vi "run.vi"(7 "abortEvent":refnum<user-event>, 8 "error in (no error)":errorcluster, 10 "TestResult in":refnum<class "TestResult.lvclass">, 11 "TestSuite in":refnum<class "TestSuite.lvclass">) -> (0 "error out":errorcluster, 2 "TestResult out":refnum<class "TestResult.lvclass">, 3 "TestSuite out":refnum<class "TestSuite.lvclass">)   [LabVIEW 2013, in "TestSuite.lvclass"]
uses:
  TestSuite.lvclass
  TestResult/TestResult.lvclass
  TestSuite.lvclass/TestSuite.ctl
  Method--enum.ctl
  suiteStatusChanged--Cluster.ctl
  suiteStatus--enum.ctl
  TestCase/TestCase.lvclass
  Libraries/VITesterUtilities.lvlib
panel:
  # "JKI VI Tester for LabVIEW\nhttp://jkisoft.com/vi-tester\nCopyright (C) 2007-2009, JKI <info@jkisoft.com>\nALL RIGHTS RESERVED"
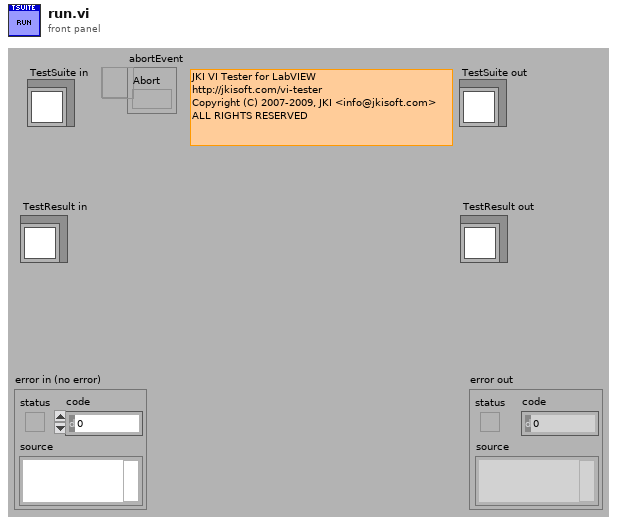
[diagram p1: front panel]
types:
  T1 = typedef "TestSuite.lvclass/suiteStatusChanged--Cluster.ctl" = cluster{"TestSuite":refnum<class>, "suiteStatus":T2}
  T2 = typedef "TestSuite.lvclass/suiteStatus--enum.ctl" = enum16{"suiteStart", "suiteStop", "suiteSkip"}
  T3 = typedef "TestSuite.lvclass/Method--enum.ctl" = enum16{"setUp", "tearDown"}
  T4 = typedef "TestResult.lvclass/shouldStop.ctl" = bool
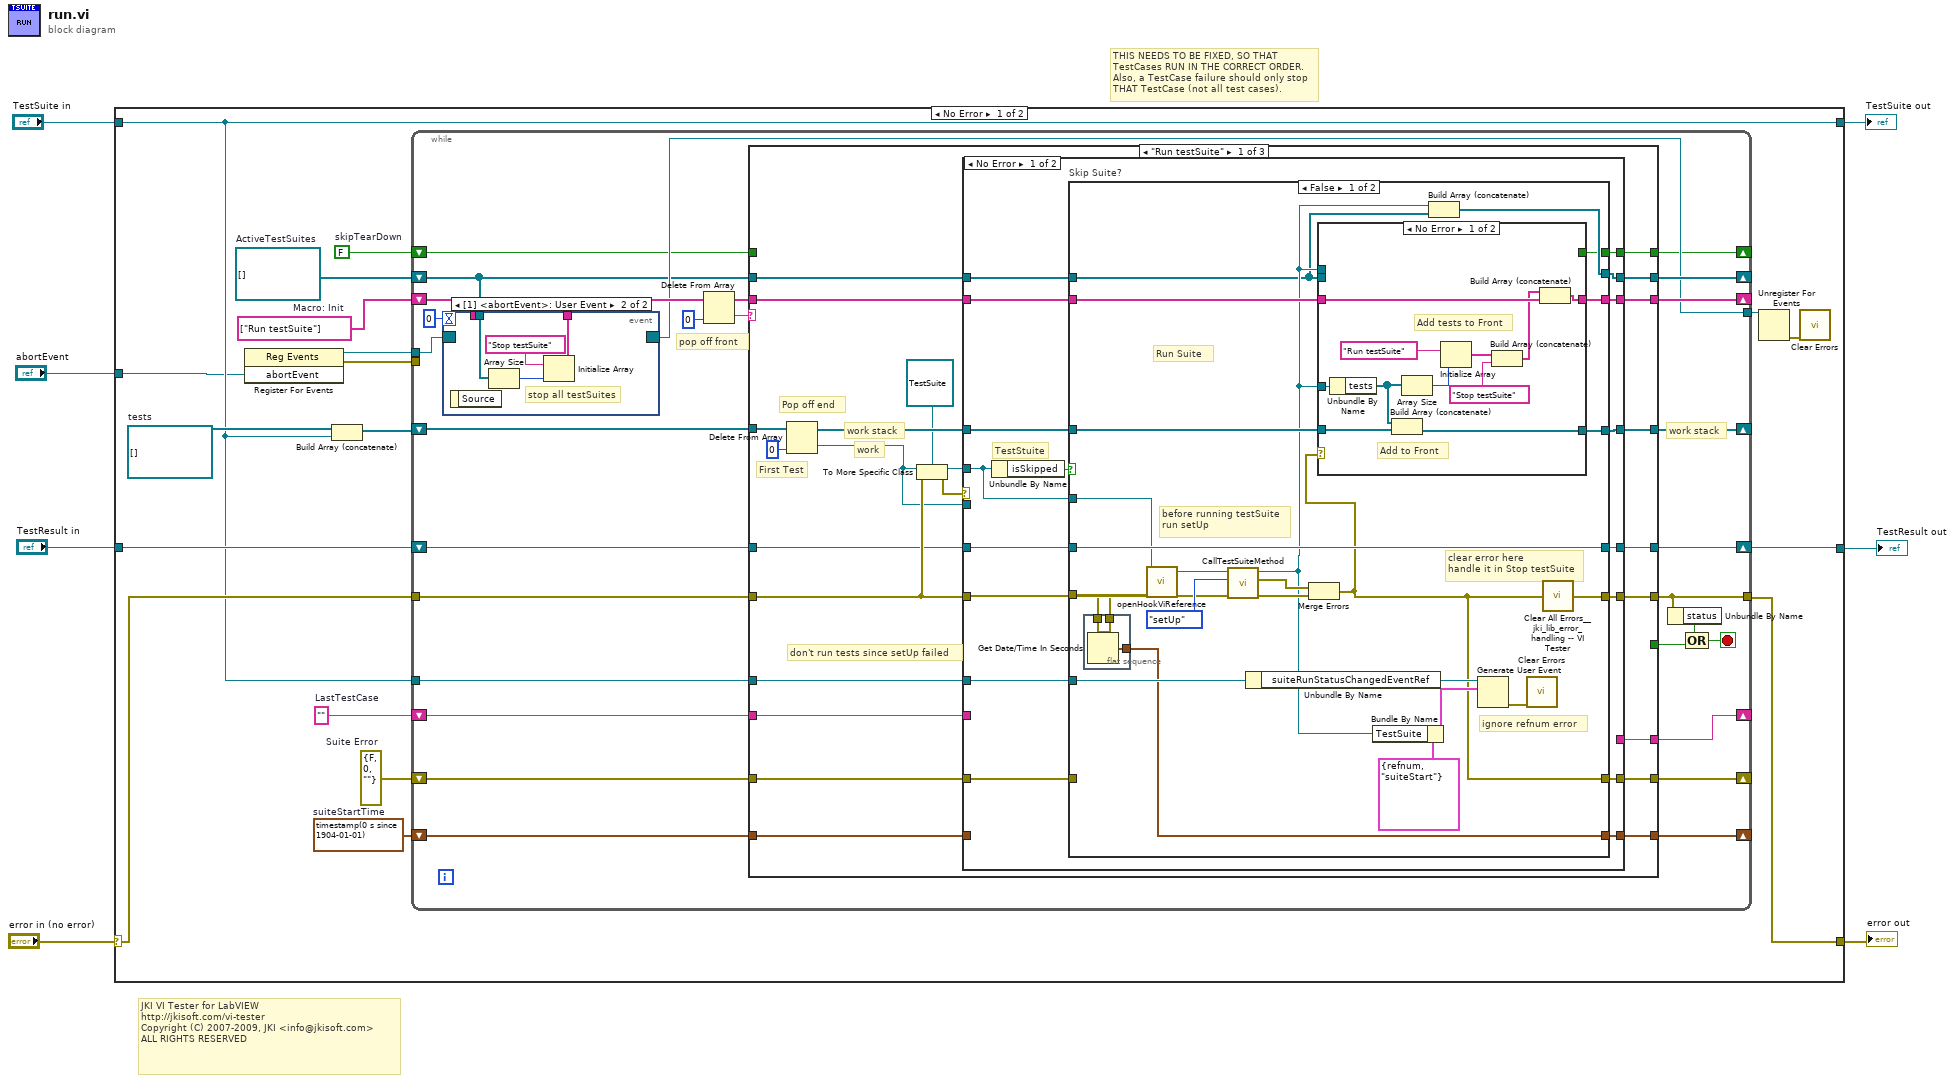
[diagram p0: block diagram]
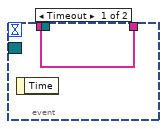
[diagram p2: hidden frame]
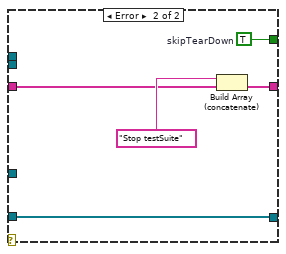
[diagram p3: hidden frame]
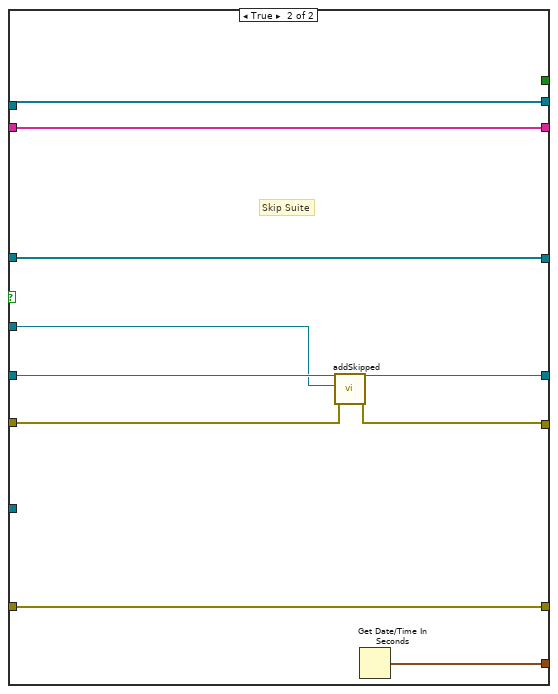
[diagram p4: hidden frame]
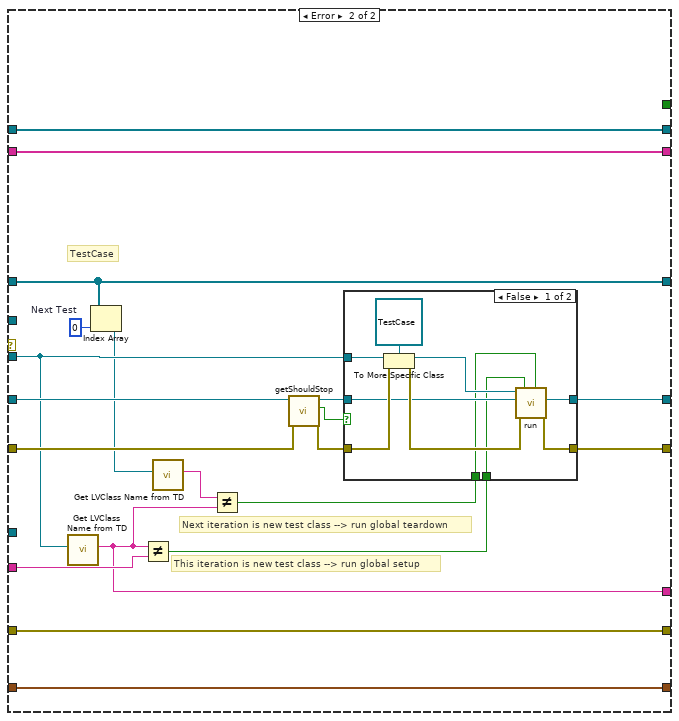
[diagram p5: hidden frame]
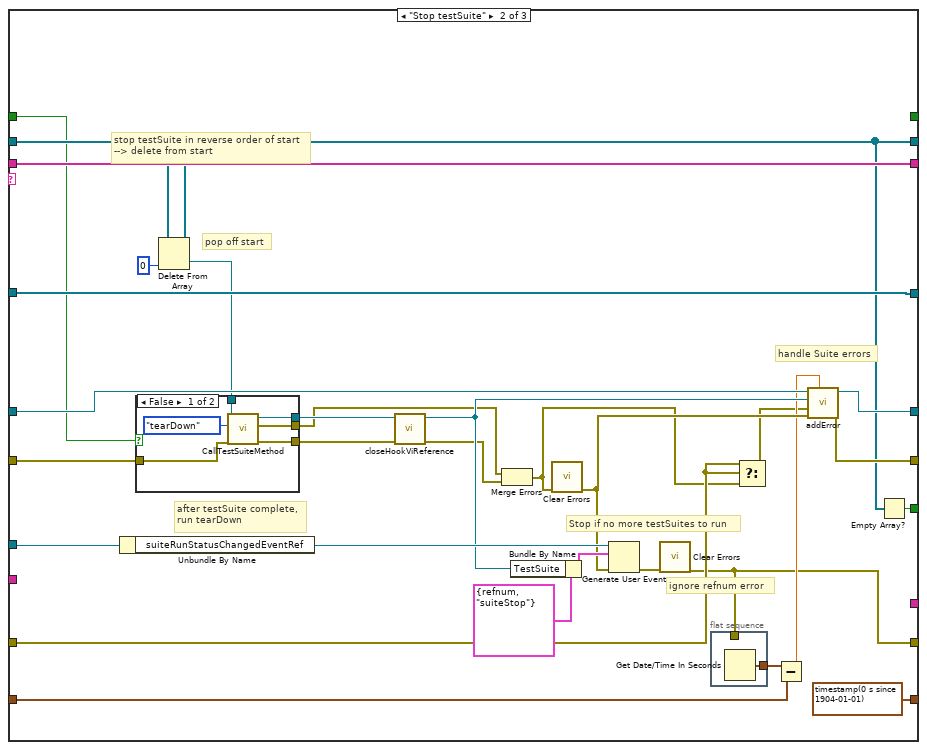
[diagram p7: hidden frame]
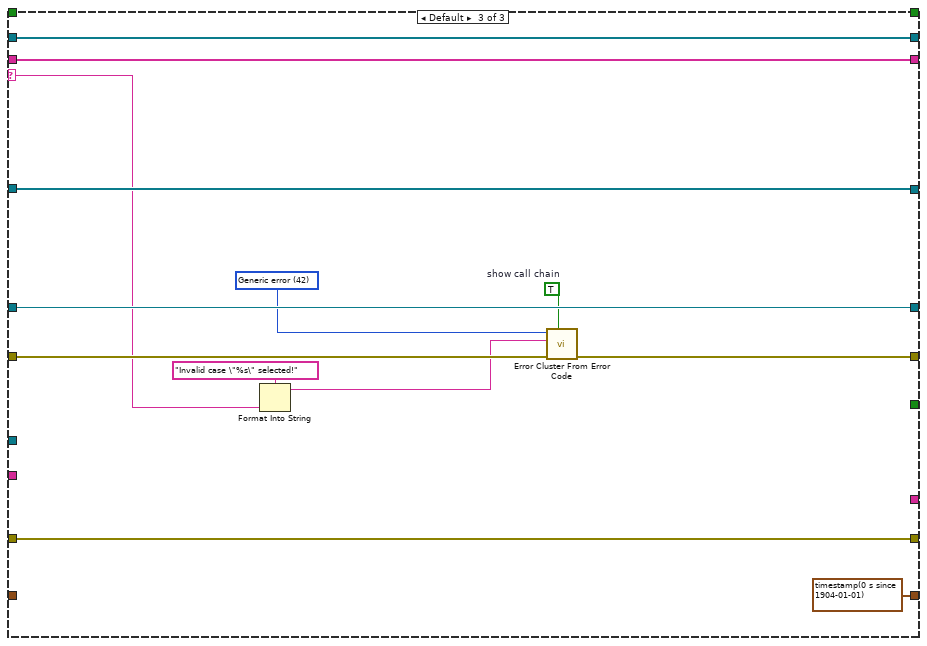
[diagram p9: hidden frame]
diagram:
  # "JKI VI Tester for LabVIEW\nhttp://jkisoft.com/vi-tester\nCopyright (C) 2007-2009, JKI <info@jkisoft.com>\nALL RIGHTS RESERVED"
  # "THIS NEEDS TO BE FIXED, SO THAT TestCases RUN IN THE CORRECT ORDER.  Also, a TestCase failure should only stop THAT TestCase (not all test cases)."
  n1 = case shown="No Error" "error in (no error)" {
    selector: "error in (no error)" -> [w21 w241]
    tunnel: [w20 w241] -> w6
    tunnel: [w17 w240] -> w4
    tunnel: "TestSuite in" -> [w17 w240]
    tunnel: "TestResult in" -> [w22 w239]
    tunnel: [w19 w239] -> w2
    tunnel: "abortEvent" -> [w16 _]
    frame No Error {
      w8 = ""  # LastTestCase
      w9 = errorcluster {"status"=FALSE, "code"=0, "source"=""}  # Suite Error
      w10 = timestamp(0 s since 1904-01-01)  # suiteStartTime
      w18 = string[] ["Run testSuite"]  # Macro: Init
      w24 = refnum<class>[] []  # tests
      w25 = refnum<class "TestSuite.lvclass">[] []  # ActiveTestSuites
      w11 = FALSE  # skipTearDown
      n2 = register-events(w16) -> (reference out=w14:refnum<event-registration>, error out=w15:errorcluster)  [unwired: 2 in]
      n3 = Build Array (concatenate)(w24, w17) -> (w23:refnum<class>[])
      n4 = while {
        tunnel: w21 -> [w54]
        tunnel: [w35] -> w20
        shift-right: [w52] -> _
        shift-left: w23 -> [w53]
        shift-right: [w51] -> w19
        shift-left: w22 -> [w50]
        shift-right: [w47] -> _
        shift-left: w18 -> [w41]
        shift-right: [w46] -> _
        shift-left: w25 -> [w38]
        tunnel: w17 -> [w44]
        tunnel: w15 -> [_]
        tunnel: w14 -> [w43]
        tunnel: [w39] -> w13
        shift-right: [w37] -> _
        shift-left: w11 -> [w36]
        shift-right: [w31] -> _
        shift-left: w10 -> [w30]
        shift-right: [w28] -> _
        shift-left: w9 -> [w29]
        shift-right: [w26] -> _
        shift-left: w8 -> [w27]
        stop <- w32 stop-if-true
        # "pop off front"
        # "work stack"
        n5 = event shown="[1] <abortEvent>: User Event" {
          selector: w43 -> [_ _]
          dyn-events: [_ _] -> w39
          timeout: 0 -> [_ _]
          tunnel: w41 -> [w55 _]
          tunnel: [w55 w56] -> w40
          tunnel: w38 -> [_ w57]
          event Timeout {
            n6 = event-data() -> ()  [unwired: 1 in, 1 out]
          }
          event User Event {
            # "stop all testSuites"
            n7 = event-data() -> ()  [unwired: 1 in, 1 out]
            n8 = Array Size(array=w57) -> (size(s)=w58:i32)
            n9 = Initialize Array("Stop testSuite", w58) -> (w56:string[])
          }
        }
        n10 = Delete From Array(array=w40, index=0) -> (deleted portion=w49:string, array with subset deleted=w48:string[])  [unwired: 1 in]
        n11 = case "TestSuite Action" shown="\"Run testSuite\"" w49 {
          selector: w49 -> [_ _ w231]
          tunnel: w54 -> [w83 w215 w233]
          tunnel: [w82 w214 w232] -> w35
          tunnel: w53 -> [w81 w212 w236]
          tunnel: [w78 w212 w236] -> w52
          tunnel: [w77 w213 w235] -> w51
          tunnel: w50 -> [w76 w216 w235]
          tunnel: w38 -> [w69 w210 w238]
          tunnel: w48 -> [w70 w211 w237]
          tunnel: [w71 w211 w237] -> w47
          tunnel: [w68 w207 w238] -> w46
          tunnel: [_ w208 _] -> w33
          tunnel: w44 -> [w67 w203 _]
          tunnel: w36 -> [_ w194 _]
          tunnel: [w66 _ _] -> w37
          tunnel: [w65 timestamp(0 s since 1904-01-01) ("suiteStartTime") timestamp(0 s since 1904-01-01) ("suiteStartTime")] -> w31
          tunnel: w30 -> [w64 w192 _]
          tunnel: w29 -> [w63 w189 w226]
          tunnel: [w62 w186 w226] -> w28
          tunnel: w27 -> [w61 _ _]
          tunnel: [w60 _ _] -> w26
          frame "Run testSuite" {
            # "don't run tests since setUp failed"
            # "First Test"
            # "Pop off end"
            # "work"
            # "work stack"
            n12 = Delete From Array(array=w81, index=0) -> (deleted portion=w80:refnum<class>, array with subset deleted=w79:refnum<class>[])  [unwired: 1 in]
            n13 = To More Specific Class(target class=refnum<class "TestSuite.lvclass"> refnum ("TestSuite out"), reference=w80, error in=w83) -> (specific class reference=w73:refnum<class "TestSuite.lvclass">, error out=w74:errorcluster)
            n14 = case shown="No Error" w74 {
              tunnel: [w96 w172] -> w77
              tunnel: [w97 w173] -> w82
              tunnel: w80 -> [_ w158]
              tunnel: w83 -> [w90 w169]
              tunnel: [w99 w160] -> w78
              tunnel: w79 -> [w100 w160]
              tunnel: w73 -> [w89 _]
              tunnel: w76 -> [w98 w171]
              tunnel: [w94 w166] -> w71
              tunnel: w70 -> [w95 w166]
              tunnel: w69 -> [w93 w165]
              tunnel: [w92 w165] -> w68
              tunnel: w67 -> [w91 _]
              tunnel: [w87 _] -> w66
              tunnel: [w86 w164] -> w65
              tunnel: w64 -> [_ w164]
              tunnel: w63 -> [w85 w163]
              tunnel: [w84 w163] -> w62
              tunnel: w61 -> [_ w162]
              tunnel: [_ w154] -> w60
              frame No Error {
                # "TestStuite"
                n15 = Unbundle By Name(w89) -> ("isSkipped"=w88:bool)
                n16 = case "Skip Suite?" shown="False" w88 {
                  tunnel: w100 -> [w125 w151]
                  tunnel: [w124 w151] -> w99
                  tunnel: w98 -> [w122 w150]
                  tunnel: [w101 w147] -> w97
                  tunnel: [w122 w149] -> w96
                  tunnel: w95 -> [w111 w153]
                  tunnel: [w110 w153] -> w94
                  tunnel: w93 -> [w108 w152]
                  tunnel: [w107 w152] -> w92
                  tunnel: w91 -> [w121 _]
                  tunnel: w90 -> [w105 w146]
                  tunnel: w89 -> [w112 w148]
                  tunnel: [w106 _] -> w87
                  tunnel: [w103 w145] -> w86
                  tunnel: w85 -> [_ w144]
                  tunnel: [w102 w144] -> w84
                  frame False {
                    # "clear error here\nhandle it in Stop testSuite"
                    # "Run Suite"
                    # "ignore refnum error"
                    # "before running testSuite\nrun setUp"
                    n17 = flat-sequence {
                      tunnel: [w127] -> w104
                      tunnel: w105 -> [w127]
                      tunnel: [w126] -> w103
                      frame #0 {
                        n18 = Get Date/Time In Seconds() -> (seconds since 1Jan1904=w126:timestamp)
                      }
                    }
                    n19 = call "openHookViReference.vi"("error in (no error)"=w104, "TestSuite in"=w112) -> ("error out"=w117:errorcluster, "TestSuite out"=w116:refnum<class "TestSuite.lvclass">)  [unwired: 8 in]
                    n20 = call "CallTestSuiteMethod.vi"("error in"=w117, "method"=Method--enum."setUp", "TestSuite in"=w116) -> ("error out"=w114:errorcluster, "Test Method Error"=w115:errorcluster, "TestSuite out"=w109:refnum<class "TestSuite.lvclass">)  [unwired: 6 in]
                    n21 = Unbundle By Name(w121) -> ("suiteRunStatusChangedEventRef"=w120:refnum<user-event>)
                    n22 = Merge Errors(w115, w114) -> (w102:errorcluster)
                    n23 = case shown="No Error" w102 {
                      tunnel: w125 -> [w138 w143]
                      tunnel: [w137 w143] -> w124
                      tunnel: w109 -> [w131 _]
                      tunnel: w111 -> [w130 w141]
                      tunnel: [w128 w140] -> w110
                      tunnel: w109 -> [_ _]
                      tunnel: w108 -> [_ _]
                      tunnel: [_ w139] -> w106
                      frame No Error {
                        # "Add tests to Front"
                        # "Add to Front"
                        n24 = Unbundle By Name(w131) -> ("tests"=w135:refnum<class>[])
                        n25 = Build Array (concatenate)(w135, w138) -> (w137:refnum<class>[])
                        n26 = Array Size(array=w135) -> (size(s)=w134:i32)
                        n27 = Initialize Array("Run testSuite", w134) -> (w132:string[])
                        n28 = Build Array (concatenate)(w132, "Stop testSuite") -> (w129:string[])
                        n29 = Build Array (concatenate)(w129, w130) -> (w128:string[])
                      }
                      frame Error {
                        w139 = TRUE  # skipTearDown
                        n30 = Build Array (concatenate)("Stop testSuite", w141) -> (w140:string[])
                      }
                    }
                    n31 = Bundle By Name(cluster=T1 {"TestSuite"=refnum, "suiteStatus"=enum."suiteStart"} ("suiteStatusChanged"), "TestSuite"=w109) -> (w119:T1)
                    n32 = Build Array (concatenate)(w109, w108) -> (w107:refnum<class "TestSuite.lvclass">[])
                    n33 = Generate User Event(user event=w120, event data cluster=w119) -> (error out=w118:errorcluster)  [unwired: 2 in, 1 out]
                    n34 = call <vilib>:"Clear Errors.vi"("error in (no error)"=w118) -> ()  [unwired: 6 in, 1 out]
                    n35 = call "Clear All Errors__jki_lib_error_handling -- VI Tester.vi"("error in"=w102) -> ("no error out"=w101:errorcluster)  [unwired: 4 in]
                  }
                  frame True {
                    # "Skip Suite"
                    n36 = call-dynamic "addSkipped.vi"("error in (no error)"=w146, "test"=w148, "TestResult in"=w150) -> ("error out"=w147:errorcluster, "TestResult out"=w149:refnum<class "TestResult.lvclass">)  [unwired: 7 in]
                    n37 = Get Date/Time In Seconds() -> (seconds since 1Jan1904=w145:timestamp)
                  }
                }
              }
              frame Error {
                w159 = 0  # Next Test
                # "This iteration is new test class --> run global setup"
                # "Next iteration is new test class --> run global teardown"
                # "TestCase"
                n38 = call "Get LVClass Name from TD.vi"("Variant"=w158) -> ("LVClass Name"=w154:string)  [unwired: 9 in, 1 out]
                n39 = Index Array(array=w160, index=w159) -> (element=w157:refnum<class>)
                n40 = Not Equal?(x=w154, y=w162) -> (x != y?=w161:bool)
                n41 = call "Get LVClass Name from TD.vi"("Variant"=w157) -> ("LVClass Name"=w156:string)  [unwired: 9 in, 1 out]
                n42 = Not Equal?(x=w156, y=w154) -> (x != y?=w155:bool)
                n43 = call-dynamic "getShouldStop.vi"("error in (no error)"=w169, "TestResult in"=w171) -> ("error out"=w168:errorcluster, "shouldStop"=w167:T4, "TestResult out"=w170:refnum<class "TestResult.lvclass">)  [unwired: 7 in]
                n44 = case shown="False" w167 {
                  tunnel: w158 -> [w182 _]
                  tunnel: [w181 w184] -> w173
                  tunnel: [w180 w185] -> w172
                  tunnel: w170 -> [w176 w185]
                  tunnel: w168 -> [w179 w184]
                  tunnel: w161 -> [w175 _]
                  tunnel: w155 -> [w174 _]
                  frame False {
                    n45 = To More Specific Class(target class=refnum<class "TestCase.lvclass"> refnum ("reference in"), reference=w182, error in=w179) -> (specific class reference=w178:refnum<class "TestCase.lvclass">, error out=w177:errorcluster)
                    n46 = call "run.vi"("RunGlobalTearDown"=w174, "RunGlobalSetup"=w175, "error in (no error)"=w177, "TestResult in (None: Create New)"=w176, "TestCase in"=w178) -> ("error out"=w181:errorcluster, "TestResult out"=w180:refnum<class "TestResult.lvclass">)  [unwired: 4 in, 1 out]
                  }
                  frame True {
                  }
                }
              }
            }
          }
          frame "Stop testSuite" {
            # "handle Suite errors"
            # "ignore refnum error"
            # "pop off start"
            # "Stop if no more testSuites to run"
            # "stop testSuite in reverse order of start\n--> delete from start"
            # "after testSuite complete,\nrun tearDown"
            n47 = Unbundle By Name(w203) -> ("suiteRunStatusChangedEventRef"=w206:refnum<user-event>)
            n48 = Delete From Array(array=w210, index=0) -> (deleted portion=w209:refnum<class "TestSuite.lvclass">, array with subset deleted=w207:refnum<class "TestSuite.lvclass">[])  [unwired: 1 in]
            n49 = case shown="False" w194 {
              tunnel: w215 -> [w222 w225]
              tunnel: w209 -> [w221 w224]
              tunnel: [w220 w224] -> w201
              tunnel: [w219 w225] -> w199
              tunnel: [w218 w225] -> w198
              frame False {
                n50 = call "CallTestSuiteMethod.vi"("error in"=w222, "method"=Method--enum."tearDown", "TestSuite in"=w221) -> ("error out"=w219:errorcluster, "Test Method Error"=w218:errorcluster, "TestSuite out"=w220:refnum<class "TestSuite.lvclass">)  [unwired: 6 in]
              }
              frame True {
              }
            }
            n51 = call "closeHookViReference.vi"("error in (no error)"=w199, "TestSuite in"=w201) -> ("error out"=w197:errorcluster, "TestSuite out"=w200:refnum<class "TestSuite.lvclass">)  [unwired: 8 in]
            n52 = Merge Errors(w198, w197) -> (w188:errorcluster)
            n53 = Bundle By Name(cluster=T1 {"TestSuite"=refnum, "suiteStatus"=enum."suiteStop"} ("suiteStatusChanged"), "TestSuite"=w200) -> (w205:T1)
            n54 = call <vilib>:"Clear Errors.vi"("error in (no error)"=w188) -> ("error out"=w196:errorcluster)  [unwired: 6 in]
            n55 = Generate User Event(user event=w206, event data cluster=w205, error in=w196) -> (error out=w204:errorcluster)  [unwired: 1 in, 1 out]
            n56 = call <vilib>:"Clear Errors.vi"("error in (no error)"=w204) -> ("error out"=w186:errorcluster)  [unwired: 6 in]
            n57 = flat-sequence {
              tunnel: w186 -> [_]
              tunnel: [w217] -> w193
              frame #0 {
                n58 = Get Date/Time In Seconds() -> (seconds since 1Jan1904=w217:timestamp)
              }
            }
            n59 = Select(t=w189, s=w189, f=w188) -> (s? t:f=w187:errorcluster)
            n60 = Subtract(x=w193, y=w192) -> (x-y=w191:dbl)
            n61 = call-dynamic "addError.vi"("execution time (sec)"=w191, "error in (no error)"=w196, "test error"=w187, "test"=w200, "TestResult in"=w216) -> ("error out"=w214:errorcluster, "TestResult out"=w213:refnum<class "TestResult.lvclass">)  [unwired: 5 in]
            n62 = Empty Array?(array=w207) -> (empty?=w208:bool)
          }
          frame Default {
            w228 = TRUE  # show call chain
            w234 = 42 items=["No error", "Argument error", "Memory is full", "Out of zone", "End of file", "File already open", "Generic file I/O error", "File not found", "File permission error", "Disk is full", "Duplicate path", "Too many files open", "System feature not enabled", "Resource file not found", "Cannot add resource", "Resource not found", "Image not found", "Image memory error", "Pen does not exist", "Config type invalid", "Config token not found", "Config parse error", "Config memory error", "Bad external code format", "Bad external code offset", "External code not present", "Null window", "Destroy window error", "Null menu", "Print aborted", "Bad print record", "Print driver error", "Windows error during printing", "Memory error during printing", "Print dialog error", "Generic print error", "Invalid device refnum", "Device not found", "Device parameter error", "Device unit error", "Cannot open device", "Device call aborted", "Generic error", "Cancelled by user", "Object ID too low", "Object ID too high", "Object not in heap", "Unknown heap", "Unknown object (invalid DefProc)", "Unknown object (DefProc not in table)", "Message out of range", "Invalid (null) method", "Unknown message", "Manager call not supported", "Bad address", "Network operation in progress", "Network operation timed out", "Connection is busy", "Network attribute not supported", "Network error", "Address in use", "System out of memory", "Connection aborted", "Connection refused", "Not connected", "Already connected", "Connection closed", "Initialization error (interapplication manager)", "Bad occurrence", "Wait on unbound occurrence handler", "Occurrence queue overflow", "Datalog type conflict", "Unused", "Unrecognized type (interapplication manager)", "Memory corrupt", "Failed to make temporary DLL", "Old CIN version", "Drag socket not found", "Failed to load drop-object", "Failed to register OLE object", "Failed to release OLE object", "Format specifier type mismatch", "Unknown format specifier", "Too few format specifiers", "Too many format specifiers", "Scan failed", "Newer CIN version", "Error converting to variant", "Runtime menu error", "Password tampered", "Variant attribute not found", "Incompatible variant data type", "Event data is not available", "Event Store is not present", "Occurrence is not found", "Event Queue is not created", "Event info is not available", "Refnum passed is NULL", "Error retrieving Class GUID", "Error retrieving CoClass GUID", "Error retrieving TypeLib GUID.", "Bad built application magic bytes.", "Specific driver is different from the specific driver associated with the Logical Name.", "There is no session opened to the class driver.", "Max Error", "MAX - Error with config objects", "MAX - Error loading configuration", "MAX - Group not supported"]
            n63 = Format Into String(format string="Invalid case \"%s\" selected!", w231) -> (resulting string=w229:string)  [unwired: 2 in, 1 out]
            n64 = call <vilib>:"Error Cluster From Error Code.vi"("show call chain? (False)"=w228, "error in (no error)"=w233, "error message (\"\")"=w229, "error code (0)"=w234) -> ("error out"=w232:errorcluster)  [unwired: 5 in]
          }
        }
        n65 = Unbundle By Name(w35) -> ("status"=w34:bool)
        n66 = Compound Arithmetic op=OR(w34, w33) -> (w32:bool)
      }
      n67 = Unregister For Events(event registration refnum=w13) -> (error out=w12:errorcluster)  [unwired: 1 in]
      n68 = call <vilib>:"Clear Errors.vi"("error in (no error)"=w12) -> ()  [unwired: 6 in, 1 out]
    }
    frame Error {
    }
  }
  "error out" <- w6
  "TestSuite out" <- w4
  "TestResult out" <- w2
